vi "Tetra_RX-PROD_Setup.vi"() -> (0 "error out":errorcluster, 2 "Status":string)   [LabVIEW 2018]
uses:
  <vilib>/Utility/error.llb/DialogType.ctl
  Initialize References/Sequence Globals.vi
  Tetra_Globals.vi
  Infrastructure/Test Parameter Globals_1.0.0.vi
  Initialize References/Station References Global.vi
  Infrastructure/Test Result File Name Global.vi
  <vilib>/Utility/file.llb/Write Delimited Spreadsheet (DBL).vi
  <vilib>/Utility/error.llb/Error Cluster From Error Code.vi
  <vilib>/Utility/file.llb/Read Delimited Spreadsheet (string).vi
  <vilib>/Utility/file.llb/Write Delimited Spreadsheet (string).vi
  <vilib>/ErrorRing/Error Ring.xnode
  Instruments/PNA/lib functions/Agilent ENA Series.lvlib
  Instruments/Agilent N5232A PNA-L/Labview Driver/Keysight PNA Series/Keysight PNA Series.lvlib
  Instruments/Agilent PSG MXG Series/Agilent PSG MXG Series.lvlib
panel:
  in  "RevBTestBoard(t)":bool=TRUE
  out "RF_CAL_PATH(str)":string
  out "Capt_Rx_Data(t)":bool
  out "capt_dir":string
  out "Pmic_FwRev":string
  out "snic":string="#Family: 0x2D\n#Serial: 0x000036092740\r\n"
  out "rev":string="rdiv\r\n0)  sw3p6:   195 mA  3616 mV\r\n1)  sw5p5:    89 mA  5472 mV\r\n2) sw2p8a:   315 mA  2784 mV\r\n3) sw2p8b:   349 mA  2768 mV\r\n4)  sw2p4:  1458 mA  2288 mV\r\n5)  sw1p4:  1047 mA  1304 mV\r\n>"
  out "Tab Control":enum32{"Page 1", "Page 2", "Page 3", "Page 4"}(tab)
  in  "Setup Chip (T)":bool=TRUE
  in  "Setup Power Supply (T)":bool=TRUE
  in  "Setup PNA (T)":bool=TRUE
  in  "Kill Teraterm":bool=TRUE
  in  "Setup Gantry(t)":bool=TRUE
  out "FPGA_Booted":bool
  out "CAL_ADC(t)":bool
  out "Ping_Success":bool
  out "Success":bool
  out "COM PORT":string
  out "adccal":string
  out "fixed_if(t)":bool=TRUE
  out "Apply_FSPL":bool
  out "Use PS1-1":bool=TRUE
  out "Temp(t)":bool=TRUE
  out "FAST_DATA":bool
  out "IF_FREQ_MHZ":dbl caption="Delay Time (s)"
  out "MODE":string
  out "Text":refnum<vi>
  out "RF_POWER":dbl
  out "RF_FREQ":dbl
  out "REF_PWR":dbl
  out "REF_FREQ":dbl
  out "RX_GAIN":i32
  out "PS1-1(V)":dbl=3.0
  out "PS1-1(A)":dbl
  out "Array":dbl[][](array[numeric])
  out "RX_N_FREQ_LIST":dbl[](array[numeric])
  out "Temp Soak(min)":dbl caption="Delay Time (s)"
  out "Gantry_Z":dbl
  out "PORT":i16
  out "i_mon":string
  out "CMD":string
  out "fspl_cal_file":path
  out "PNA_STATE":string
  out "FSPL_CAL_FILE_DIR":path=path "C:/RageATE/Automated Tests/Tetra WAM/DVT/Cal Files/FSPL.csv"
  out "RF_CAL_PATH":path
  out "HORN_CAL_PATH":path
  out "NF_SPEC_FILE":path
  out "git log":string="#RageATE gitlog: commit 3f967c02fb9022fedaa326db1cba8dee33b37288\n#RageATE gitlog: Author: Rick-Rage <74794943+Rick-Rage@users.noreply.github.com>\n#RageATE gitlog: Date:   Tue Nov 23 14:33:10 2021 -0500\n#RageATE gitlog: This Computer Name : CRANES\r\n\r\n"
  out "TEMP":dbl=4.75
  out "Use PS1-2":bool=TRUE
  out "PS1-2(A)":dbl
  out "PS1-2(V)":dbl=1000000.0
  in  "error in (no error)":errorcluster
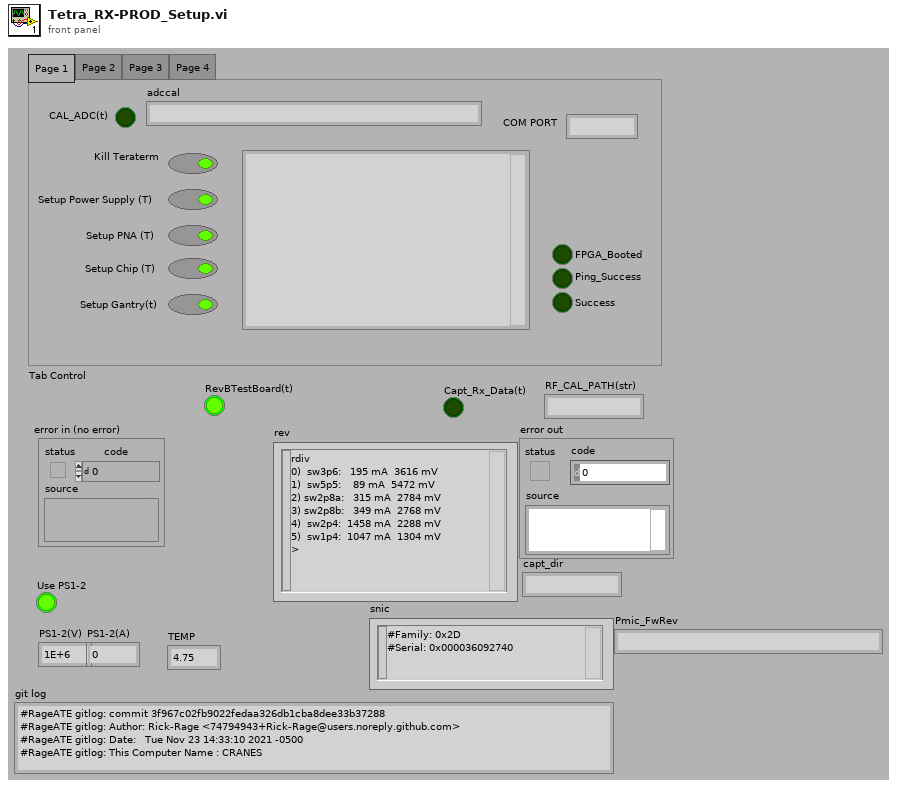
[diagram p1: front panel]
types:
  T1 = typedef "DialogType.ctl" = u16
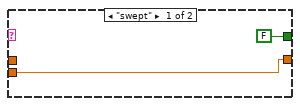
[diagram p4: hidden frame]
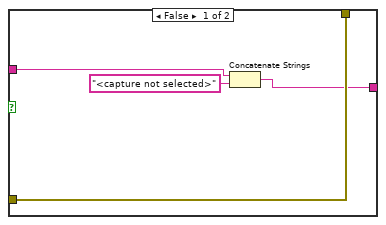
[diagram p5: hidden frame]
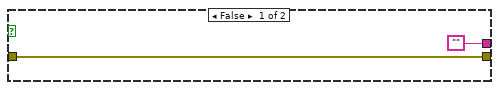
[diagram p6: hidden frame]
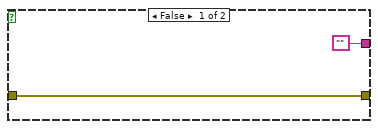
[diagram p7: hidden frame]
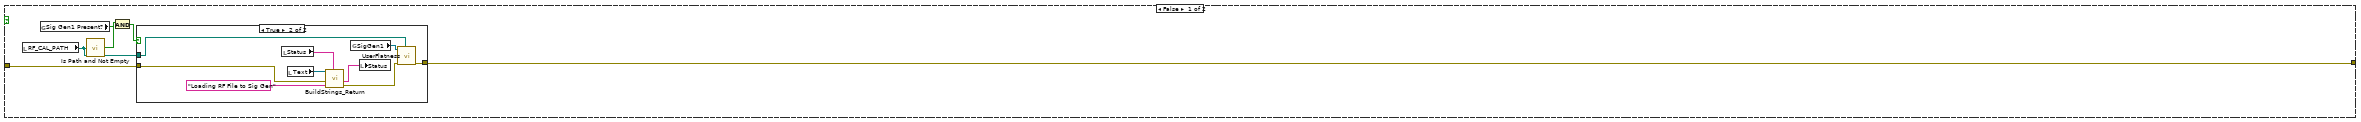
[diagram p8: hidden frame]
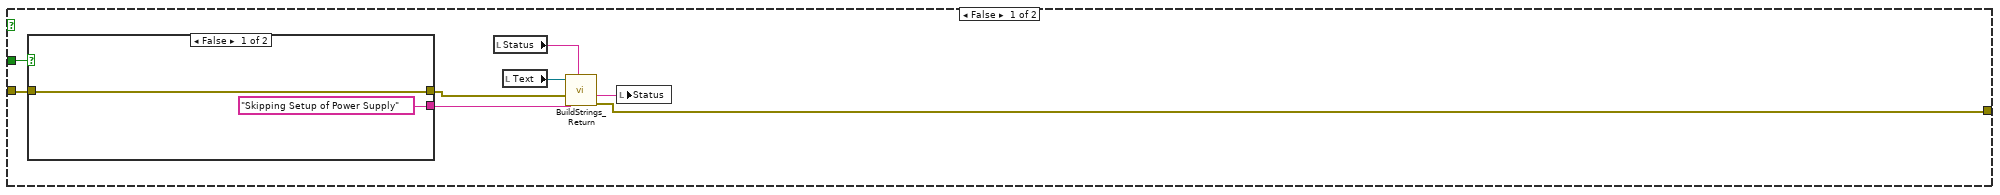
[diagram p15: hidden frame]
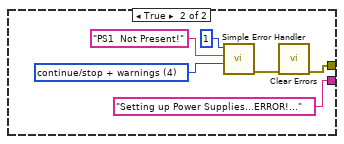
[diagram p16: hidden frame]
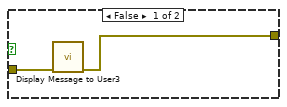
[diagram p18: hidden frame]
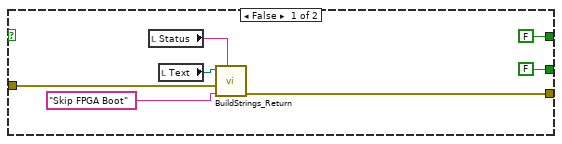
[diagram p20: hidden frame]
diagram:
  n1 = flat-sequence {
    tunnel: [w38] -> w18
    tunnel: w18 -> [w71]
    tunnel: [w70] -> w17
    tunnel: [w69] -> w16
    tunnel: [w67] -> w7
    tunnel: [w101] -> w9
    tunnel: w17 -> [w150]
    tunnel: w16 -> [w149]
    tunnel: w7 -> [w101]
    tunnel: w9 -> [w167]
    tunnel: [w177] -> w8
    tunnel: w8 -> [w229]
    tunnel: [w228] -> w14
    tunnel: w14 -> [w377]
    tunnel: [w376] -> w13
    tunnel: w13 -> [w385]
    tunnel: [w385] -> w1
    tunnel: [w387] -> w11
    tunnel: w1 -> [w386]
    tunnel: w11 -> [w473]
    tunnel: [w472] -> w4
    tunnel: [w510] -> w5
    tunnel: w4 -> [w509]
    tunnel: [w558] -> w6
    tunnel: w5 -> [w557]
    tunnel: w6 -> [w585]
    tunnel: [w584] -> w10
    tunnel: [w642] -> w19
    tunnel: w10 -> [w632]
    tunnel: [w794] -> w15
    tunnel: w19 -> [w788]
    tunnel: w15 -> [w838]
    tunnel: [w837] -> w3
    tunnel: w3 -> [w861]
    tunnel: [w860] -> w2
    tunnel: [w905] -> w12
    tunnel: w2 -> [w916]
    frame #0 {
      w28 = FALSE ("FPGA_Booted")
      # "Kill TeraTerm"
      n2 = flat-sequence {
        tunnel: [w57] -> w20
        tunnel: [w47] -> w21
        frame #0 {
          w54 = 0 items=["INPUT", "OUTPUT"] ("line index")
          # "C:\\RageATE\\Automated Tests\\Tetra WAM\\Support"
          n3 = global read "Sequence Globals.vi" "DevSupportPath"() -> (w44:path)
          n4 = Strip Path(path=w44) -> (stripped path=w43:path)  [unwired: 1 out]
          n5 = global read "Sequence Globals.vi" "AppSupportPath"() -> (w52:path)
          n6 = Build Path(base path=w43, name or relative path=path "Automated Tests/Tetra WAM/PRODUCTION/Test Benches" ("base path")) -> (appended path=w41:path)
          n7 = global read "Tetra_Globals.vi" "TestBench_ID"() -> (w45:string)
          n8 = global read "Sequence Globals.vi" "IsRuntime?"() -> (w40:bool)
          n9 = Build Path(base path=w41, name or relative path=w45) -> (appended path=w56:path)
          n10 = Concatenate Strings(w45, " Calibration Files" ("name or relative path")) -> (w46:string)
          n11 = Build Path(base path=w56, name or relative path=w46) -> (appended path=w53:path)
          n12 = Select(t=w52, s=w40, f=w53) -> (s? t:f=w48:path)
          n13 = call "FindMostRecentCalFile.vi"("DIR_IN"=w48, "Test Bench (for filename match)"=w45, "line index"=w54, "IsRuntime?"=w40) -> ("Success?(t)"=w50:bool, "cal_path_out"=w51:path)  [unwired: 9 in, 1 out]
          n14 = case shown="False" w50 {
            tunnel: [path "" ("appended path") w60] -> w57
            tunnel: w51 -> [_ w60]
            frame False {
              n15 = Two Button Dialog(message="There Are No INPUT cal files") -> ()  [unwired: 2 in, 1 out]
            }
            frame True {
            }
          }
          n16 = Build Path(base path=w48, name or relative path="FSPL.csv") -> (appended path=w47:path)
        }
      }
      n17 = global read "Sequence Globals.vi" "RageATE_Gitlog"() -> (→"git log":string)
      n18 = local write "RevBTestBoard(t)"("RevBTestBoard(t)") -> ()
      n19 = local write "CAL_ADC(t)"(w28) -> ()
      n20 = local write "Setup PNA (T)"("Setup PNA (T)") -> ()
      n21 = local write "Setup Gantry(t)"("Setup Gantry(t)") -> ()
      n22 = local write "Setup Chip (T)"("Setup Chip (T)") -> ()
      n23 = local write "Setup Power Supply (T)"("Setup Power Supply (T)") -> ()
      n24 = case shown="True" "Kill Teraterm" {
        tunnel: "error in (no error)" -> [w61 w63]
        tunnel: [w61 w62] -> w38
        tunnel: "taskkill /f /im ttermpro.exe" ("command line") -> [_ w65]
        frame False {
        }
        frame True {
          n25 = call <vilib>:"Clear Errors.vi"("error in (no error)"=w63) -> ("error out"=w64:errorcluster)  [unwired: 5 in, 1 out]
          n26 = call <vilib>:"System Exec.vi"("error in (no error)"=w64, "command line"=w65) -> ("error out"=w66:errorcluster)  [unwired: 6 in, 3 out]
          n27 = call "Time Delay2"("error in (no error)"=w66) -> ("error out"=w62:errorcluster)  [unwired: 10 in]
        }
      }
      n28 = Path To String(path=w20) -> (string=w26:string)
      n29 = Concatenate Strings("#RF_Cal_Path: " ("string"), w26) -> (→"RF_CAL_PATH(str)":string)
      "Success" <- FALSE ("Success")
      "Status" <- ""
      "adccal" <- ""
      "FPGA_Booted" <- w28
      "Ping_Success" <- w28
      "Tab Control" <- enum32{"Page 1", "Page 2", "Page 3", "Page 4"}."Page 1" ("Tab Control")
      "RF_CAL_PATH" <- w20
      "FSPL_CAL_FILE_DIR" <- w21
    }
    frame #1 {
      n30 = property on="Status" class="Str"(error in=w71) -> (error out=w67:errorcluster, "Text"=→"Text":refnum<vi>)  [unwired: 1 in, 1 out]
      n31 = global read "Test Parameter Globals_1.0.0.vi" "Input Constants Out"() -> (w70:string[])
      n32 = global read "Test Parameter Globals_1.0.0.vi" "Test Parameters"() -> (w69:string[][])
    }
    frame #2 {
      w140 = 0 ("disabled index (col)")
      # "PRODUCTION\\Test Benches\\Common"
      # "PRODUCTION\\Test Benches\\Common"
      # "C:\\RageATE\\Automated Tests\\Tetra WAM\\PRODUCTION\\Test Benches\\Common\\Horn_Gain_121322.csv"
      n33 = Index Array(array=w150, index #8=12 ("index"), index #9=14 ("index"), index #11=16 ("index"), index #16=24 ("index"), index #17=10 ("index")) -> (element #1=w129:string, element #2=w122:string, element #3=w92:string, element #4=→"MODE":string, element #5=w121:string, element #6=w116:string, element #7=w151:string, element #8=→"CMD":string, element #9=→"PNA_STATE":string, element #11=w88:string, element #12=w105:string, element #13=w104:string, element #14=w103:string, element #15=w100:string, element #16=w84:string, element #17=w96:string)  [unwired: 12 in, 1 out]
      n34 = call "StringToNumberControlWithBool.vi"("String In"=w96) -> ("NOT = 0"=→"Capt_Rx_Data(t)":bool)  [unwired: 7 in, 1 out]
      n35 = Index Array(array=w149, index (row) #1=0 ("disabled index (row)"), index (col) #1=w140, index (row) #2=3 ("index (row)"), index (col) #2=w140, index (row) #3=4 ("disabled index (row)"), index (col) #3=w140, index (row) #4=7 ("disabled index (row)"), index (col) #4=w140, index (row) #5=6 ("disabled index (row)"), index (col) #5=w140) -> (element #1=w143:string, element #2=w155:string, element #3=w154:string, element #4=w145:string, element #5=w138:string)
      n36 = call "StringToNumberControlWithBool.vi"("String In"=w151) -> ("Number Out"=→"Temp Soak(min)":dbl)  [unwired: 7 in, 1 out]
      n37 = call "StringToNumberControlWithBool.vi"("String In"=w104) -> ("NOT = 0"=→"FAST_DATA":bool)  [unwired: 7 in, 1 out]
      n38 = call "StringToNumberControlWithBool.vi"("String In"=w103) -> ("NOT = 0"=→"Apply_FSPL":bool)  [unwired: 7 in, 1 out]
      n39 = call "StringToNumberControlWithBool.vi"("String In"=w100) -> ("NOT = 0"=→"CAL_ADC(t)":bool)  [unwired: 7 in, 1 out]
      n40 = call "StringToNumberControlWithBool.vi"("String In"=w155) -> ("Number Out"=→"REF_PWR":dbl)  [unwired: 7 in, 1 out]
      n41 = call "StringToNumberControlWithBool.vi"("String In"=w154) -> ("Number Out"=→"RF_POWER":dbl)  [unwired: 7 in, 1 out]
      n42 = call "StringToNumberControlWithBool.vi"("String In"=w138) -> ("Number Out"=→"RX_GAIN":dbl)  [unwired: 7 in, 1 out]
      n43 = call "StringToNumberControlWithBool.vi"("String In"=w145) -> ("Number Out"=w111:dbl)  [unwired: 7 in, 1 out]
      "RF_FREQ" <- w111
      n44 = call "StringToNumberControlWithBool(x2).vi"("string"=w129) -> ("Num(2)"=→"PS1-1(A)":dbl, "Num"=→"PS1-1(V)":dbl, "NOT_0?"=→"Use PS1-1":bool)  [unwired: 4 in, 4 out]
      n45 = call "StringToNumberControlWithBool(x2).vi"("string"=w122) -> ("Num(2)"=→"PS1-2(A)":dbl, "Num"=→"PS1-2(V)":dbl, "NOT_0?"=→"Use PS1-2":bool)  [unwired: 4 in, 4 out]
      n46 = call "TempControlWithBool.vi"("INPUT"=w143) -> ("out"=→"TEMP":dbl, "Valid(t)"=w141:bool)  [unwired: 6 in, 1 out]
      "Temp(t)" <- w141
      n47 = call "StringToNumberControlWithBool(x2).vi"("string"=w121) -> ("Num(2)"=→"Gantry_Z":dbl, "Num"=→"PORT":dbl, "NOT_0(2)"=w119:bool, "NOT_0?"=w120:bool)  [unwired: 4 in, 3 out]
      n48 = call "StringToNumberControlWithBool(x2).vi"("string"=w116) -> ("Num(2)"=w113:dbl, "before substring"=w115:string)  [unwired: 4 in, 5 out]
      "IF_FREQ_MHZ" <- w113
      n49 = global write "Station References Global.vi" "Oven Present?"(w141) -> ()
      n50 = Or(x=w120, y=w119) -> (x .or. y?=w131:bool)
      n51 = call <vilib>:"Trim Whitespace.vi"("string"=w115) -> ("trimmed string"=w112:string)  [unwired: 1 in]
      n52 = Spreadsheet String To Array(delimiter (Tab)=";", format string="", spreadsheet string=w105, array type (2D Dbl)=dbl[] []) -> (array=w133:dbl[])
      "RX_N_FREQ_LIST" <- w133
      n53 = local write "Setup Gantry(t)"(w131) -> ()
      n54 = global write "Tetra_Globals.vi" "RX_N_FREQ_LIST"(w133) -> ()
      n55 = case shown="\"fixed\", Default" w112 {
        tunnel: [FALSE ("fixed_if(t)") TRUE ("fixed_if(t)")] -> w114
        tunnel: w113 -> [_ w164]
        tunnel: w111 -> [w157 w161]
        tunnel: [w157 w159] -> w110
        frame "swept" {
        }
        frame "fixed", Default {
          n56 = Divide(x=w164, y=1000.0) -> (x/y=w160:dbl)
          n57 = Add(x=w160, y=w161) -> (x+y=w163:dbl)
          n58 = Divide(x=w163, y=2.0) -> (x/y=w159:dbl)
        }
      }
      "REF_FREQ" <- w110
      "fixed_if(t)" <- w114
      n59 = global read "Sequence Globals.vi" "AppSupportPath"() -> (w81:path)
      n60 = global read "Sequence Globals.vi" "IsRuntime?"() -> (w83:bool)
      n61 = global read "Sequence Globals.vi" "DevSupportPath"() -> (w80:path)
      n62 = String To Path(string=w84) -> (path=w85:path)
      n63 = global read "Tetra_Globals.vi" "comport"() -> (w91:refnum<visa-resource-name>)
      n64 = Empty String/Path?(string/path=w92) -> (empty?=w94:bool)
      n65 = String To Path(string=w88) -> (path=w90:path)
      n66 = Strip Path(path=w85) -> (name=w76:string)  [unwired: 1 out]
      n67 = Strip Path(path=w80) -> (stripped path=w79:path)  [unwired: 1 out]
      n68 = Select(t=w91, s=w94, f=w92) -> (s? t:f=→"COM PORT":refnum<visa-resource-name>)
      n69 = Strip Path(path=w90) -> (name=w77:string)  [unwired: 1 out]
      n70 = Build Path(base path=w81, name or relative path=w76) -> (appended path=w86:path)
      n71 = Build Path(base path=w79, name or relative path="Automated Tests\\Tetra WAM\\PRODUCTION\\setup files") -> (appended path=w72:path)
      n72 = Build Path(base path=w72, name or relative path=w77) -> (appended path=w78:path)
      n73 = Build Path(base path=w81, name or relative path=w77) -> (appended path=w89:path)
      n74 = Select(t=w89, s=w83, f=w78) -> (s? t:f=→"HORN_CAL_PATH":path)
      n75 = Build Path(base path=w72, name or relative path=w76) -> (appended path=w75:path)
      n76 = Select(t=w86, s=w83, f=w75) -> (s? t:f=→"NF_SPEC_FILE":path)
    }
    frame #3 {
      # "Shut Off Equipments Power FOR ADC CAL"
      n77 = global read "Station References Global.vi" "PNA Present?"() -> (w176:bool)
      n78 = local read "CAL_ADC(t)"() -> (w171:bool)
      n79 = And(x=w176, y=w171) -> (x .and. y?=w172:bool)
      n80 = case shown="True" w172 {
        tunnel: [w199 w205] -> w178
        tunnel: w168 -> [w199 w207]
        tunnel: ["" w200] -> w173
        frame False {
        }
        frame True {
          w208 = 3 items=["HOLD", "CONT", "GROUP", "SINGLE"] ("Mode")
          w210 = 0 items=["OFF", "ON"] ("STATE(0=OFF)")
          n81 = global read "Station References Global.vi" "PNA"() -> (w214:refnum<visa-resource-name>)
          n82 = call "PNA_MAIN_RF_STATE.vi"("Session In"=w214, "error in"=w207, "RO(T)"=FALSE, "STATE(0=OFF)"=w210) -> ("Session Out"=w213:refnum<visa-resource-name>, "error out"=w212:errorcluster)  [unwired: 9 in, 1 out]
          n83 = call "PNA_SWEEP MODE.vi"("Mode"=w208, "Channel"=1, "error in (no error)"=w212, "VISA resource name"=w213) -> ("error out"=w206:errorcluster)  [unwired: 6 in, 1 out]
          n84 = local read "Status"() -> (w204:string)
          n85 = local read "Text"() -> (w202:refnum<vi>)
          n86 = call "BuildStrings_Return.vi"("seconds to wait"=1.0, "Input String"=w204, "New String"="Shutting Off PNA Power", "error in (no error)"=w206, "reference"=w202) -> ("error out"=w205:errorcluster, "concatenated string"=w200:string)  [unwired: 4 in, 1 out]
        }
      }
      n87 = flat-sequence {
        tunnel: w167 -> [w182]
        tunnel: [w181] -> w168
        frame #0 {
          n88 = local read "Capt_Rx_Data(t)"() -> (w179:bool)
          n89 = case shown="True" w179 {
            tunnel: [w184 w196] -> w183
            tunnel: w182 -> [w187 w191]
            tunnel: [w187 w190] -> w181
            tunnel: "#CaptureFileDirectory: " ("string") -> [w186 w189]
            frame False {
              n90 = Concatenate Strings(w186, "<capture not selected>" ("string")) -> (w184:string)
            }
            frame True {
              w188 = "'" ("string")
              # "For Header"
              n91 = global read "Test Result File Name Global.vi" "Test Results File Name"() -> (w197:path)
              n92 = Path To String(path=w197) -> (string=w195:string)
              n93 = Search and Replace String(input string=w195, search string=".csv", replace string="_RxCaptureFiles.zip" ("name or relative path"), error in=w191) -> (result string=w192:string, error out=w190:errorcluster)  [unwired: 4 in, 2 out]
              n94 = Concatenate Strings(w189, w188, w192, w188) -> (w196:string)
            }
          }
          "capt_dir" <- w183
        }
      }
      n95 = global read "Station References Global.vi" "Sig Gen1 Present?"() -> (w175:bool)
      n96 = local read "CAL_ADC(t)"() -> (w169:bool)
      n97 = local write "Status"(w173) -> ()
      n98 = And(x=w169, y=w175) -> (x .and. y?=w170:bool)
      n99 = case shown="True" w170 {
        tunnel: w178 -> [w216 w224]
        tunnel: [w216 w219] -> w177
        tunnel: ["" w218] -> w174
        frame False {
        }
        frame True {
          n100 = global read "Station References Global.vi" "SigGen1"() -> (w226:refnum<visa-resource-name>)
          n101 = call "VSG_SET_RF_STATE_1.00.vi"("RF ON/OFF (OFF)"=FALSE ("Enable RF Power (T: Enable)"), "error in"=w224, "Session In"=w226) -> ("error out"=w223:errorcluster)  [unwired: 6 in, 2 out]
          n102 = local read "Status"() -> (w217:string)
          n103 = local read "Text"() -> (w222:refnum<vi>)
          n104 = call "BuildStrings_Return.vi"("seconds to wait"=2.0, "Input String"=w217, "New String"="Shutting Off SG1 Power", "error in (no error)"=w223, "reference"=w222) -> ("error out"=w219:errorcluster, "concatenated string"=w218:string)  [unwired: 4 in, 1 out]
        }
      }
      n105 = local write "Status"(w174) -> ()
    }
    frame #4 {
      n106 = local read "Apply_FSPL"() -> (w227:bool)
      n107 = case shown="True" w227 {
        tunnel: w229 -> [w231 w253]
        tunnel: [w230 w252] -> w228
        frame False {
          n108 = local read "RF_CAL_PATH"() -> (w233:path)
          n109 = global read "Station References Global.vi" "Sig Gen1 Present?"() -> (w232:bool)
          n110 = call <vilib>:"Is Path and Not Empty.vi"("path"=w233) -> ("Is Path and Not Empty?"=w234:bool)  [unwired: 4 in]
          n111 = And(x=w234, y=w232) -> (x .and. y?=w235:bool)
          n112 = case shown="True" w235 {
            tunnel: w233 -> [_ w244]
            tunnel: w231 -> [w236 w240]
            tunnel: [w236 w238] -> w230
            frame False {
            }
            frame True {
              n113 = local read "Status"() -> (w237:string)
              n114 = local read "Text"() -> (w243:refnum<vi>)
              n115 = call "BuildStrings_Return.vi"("Input String"=w237, "New String"="Loading RF File to Sig Gen", "error in (no error)"=w240, "reference"=w243) -> ("error out"=w239:errorcluster, "concatenated string"=w242:string)  [unwired: 5 in, 1 out]
              n116 = global read "Station References Global.vi" "SigGen1"() -> (w245:refnum<visa-resource-name>)
              n117 = local write "Status"(w242) -> ()
              n118 = call "UserFlatness.vi"("cal file path (dialog if empty)"=w244, "error in (no error)"=w239, "Session In"=w245) -> ("error out"=w238:errorcluster)  [unwired: 6 in, 2 out]
            }
          }
        }
        frame True {
          n119 = flat-sequence {
            tunnel: w253 -> [w346]
            tunnel: [w347] -> w254
            tunnel: w254 -> [w362]
            tunnel: [w360] -> w247
            frame #0 {
              n120 = local read "RF_CAL_PATH"() -> (w344:path)
              n121 = call <vilib>:"Is Path and Not Empty.vi"("path"=w344) -> ("Is Path and Not Empty?"=w345:bool)  [unwired: 4 in]
              n122 = case shown="True" w345 {
                tunnel: [w348 w352] -> w347
                tunnel: w344 -> [_ w355]
                tunnel: w346 -> [w348 w350]
                frame False {
                }
                frame True {
                  n123 = call "GetCalData.vi"("Open new file T"=TRUE, "error in (no error)"=w350, "DeleteHeader(t)"=TRUE, "cal file path (dialog if empty)"=w355) -> ("error out"=w351:errorcluster, "array out"=w354:dbl[][])  [unwired: 2 in, 4 out]
                  n124 = global write "Tetra_Globals.vi" "RF_CAL"(w354) -> ()
                  n125 = local read "Status"() -> (w357:string)
                  n126 = local read "Text"() -> (w359:refnum<vi>)
                  n127 = call "BuildStrings_Return.vi"("Input String"=w357, "New String"="Reading RF Cal File...", "error in (no error)"=w351, "reference"=w359) -> ("error out"=w352:errorcluster, "concatenated string"=w358:string)  [unwired: 5 in, 1 out]
                  n128 = local write "Status"(w358) -> ()
                }
              }
            }
            frame #1 {
              n129 = local read "HORN_CAL_PATH"() -> (w361:path)
              n130 = Empty String/Path?(string/path=w361) -> (empty?=w363:bool)
              n131 = case shown="False" w363 {
                tunnel: w361 -> [w374 _]
                tunnel: w362 -> [w365 w375]
                tunnel: [w368 w375] -> w360
                frame False {
                  n132 = call "GetCalData.vi"("Open new file T"=TRUE, "error in (no error)"=w365, "DeleteHeader(t)"=FALSE, "cal file path (dialog if empty)"=w374) -> ("error out"=w366:errorcluster, "array out"=w373:dbl[][])  [unwired: 2 in, 4 out]
                  n133 = global write "Tetra_Globals.vi" "HORN_CAL"(w373) -> ()
                  n134 = local read "Status"() -> (w370:string)
                  n135 = local read "Text"() -> (w372:refnum<vi>)
                  n136 = call "BuildStrings_Return.vi"("Input String"=w370, "New String"="Reading Horn Cal File...", "error in (no error)"=w366, "reference"=w372) -> ("error out"=w368:errorcluster, "concatenated string"=w371:string)  [unwired: 5 in, 1 out]
                  n137 = local write "Status"(w371) -> ()
                }
                frame True {
                }
              }
            }
          }
          n138 = flat-sequence {
            tunnel: w247 -> [w256]
            tunnel: [w255] -> w246
            frame #0 {
              n139 = local read "NF_SPEC_FILE"() -> (w257:path)
              n140 = call <vilib>:"Is Path and Not Empty.vi"("path"=w257) -> ("Is Path and Not Empty?"=w258:bool)  [unwired: 4 in]
              n141 = case shown="True" w258 {
                tunnel: w257 -> [_ w265]
                tunnel: w256 -> [w259 w262]
                tunnel: [w259 w261] -> w255
                frame False {
                }
                frame True {
                  n142 = call "GetCalData.vi"("Open new file T"=TRUE, "error in (no error)"=w262, "DeleteHeader(t)"=TRUE, "cal file path (dialog if empty)"=w265) -> ("error out"=w261:errorcluster, "array out"=w263:dbl[][])  [unwired: 2 in, 4 out]
                  n143 = global write "Tetra_Globals.vi" "NF_MASK"(w263) -> ()
                }
              }
            }
          }
          n144 = flat-sequence {
            tunnel: [w324] -> w249
            tunnel: [w313] -> w250
            tunnel: w246 -> [w312]
            frame #0 {
              n145 = global read "Tetra_Globals.vi" "HORN_CAL"() -> (w325:dbl[][])
              n146 = for {
                tunnel: w325 -> [w341] mode=indexing
                tunnel: w312 -> [w340]
                tunnel: [w331] -> w322 mode=indexing
                tunnel: [w338] -> w323
                tunnel: [w335] -> w317 mode=indexing
                tunnel: [w332] -> w315 mode=indexing
                w330 = -1.0 ("x")
                w342 = u16 2 items=["Meter", "Feet", "Inches"] ("d(units)")
                w343 = u16 0 items=["GHz", "MHz"] ("f(units)")
                # "convert to mhz"
                n147 = Index Array(array=w341) -> (element #1=w337:dbl, element #2=w339:dbl)  [unwired: 2 in]
                n148 = local read "Gantry_Z"() -> (w334:dbl)
                n149 = Multiply(x=1000.0, y=w337) -> (x*y=w335:dbl)
                n150 = call "FSPL_CALC.vi"("f"=w337, "d"=w334, "error in"=w340, "Ant1 Gain (dB)"=w339, "f(units)"=w343, "d(units)"=w342) -> ("Corr(dB)"=w329:dbl, "fsl(dB)"=w333:dbl, "error out"=w338:errorcluster)  [unwired: 11 in]
                n151 = Multiply(x=w329, y=w330) -> (x*y=w331:dbl)
                n152 = Multiply(x=w330, y=w333) -> (x*y=w332:dbl)
              }
              n153 = local read "Gantry_Z"() -> (w316:dbl)
              n154 = Number To Fractional String(number=w316) -> (F-format string=w320:string)  [unwired: 3 in]
              n155 = local read "Status"() -> (w328:string)
              n156 = Concatenate Strings("Generating FSPL Table for Z = " ("New String"), w320, " inches" ("string")) -> (w319:string)
              n157 = local read "Text"() -> (w326:refnum<vi>)
              n158 = Build Array(w317, w322, w315) -> (w314:dbl[][])
              n159 = call "BuildStrings_Return.vi"("Input String"=w328, "New String"=w319, "error in (no error)"=w323, "reference"=w326) -> ("error out"=w324:errorcluster, "concatenated string"=w327:string)  [unwired: 5 in, 1 out]
              n160 = local write "Status"(w327) -> ()
              n161 = Transpose 2D Array(2D array=w314) -> (transposed array=w313:dbl[][])
              n162 = global write "Tetra_Globals.vi" "FSPL_CAL"(w313) -> ()
            }
          }
          n163 = flat-sequence {
            tunnel: w250 -> [w269]
            tunnel: w249 -> [w268]
            tunnel: [w267] -> w248
            frame #0 {
              n164 = for {
                tunnel: w269 -> [w279] mode=indexing
                tunnel: w268 -> [w277]
                tunnel: [w276] -> w267
                tunnel: [w273] -> w266 mode=indexing
                n165 = Index Array(array=w279) -> (element #1=w278:dbl, element #2=w272:dbl)  [unwired: 2 in]
                n166 = global read "Tetra_Globals.vi" "RF_CAL"() -> (w281:dbl[][])
                n167 = call "GetCalData.vi"("Open new file T"=FALSE, "Ary In"=w281, "error in (no error)"=w277, "RF Freq (MHz)"=w278, "DeleteHeader(t)"=FALSE) -> ("error out"=w276:errorcluster, "Ampl Out"=w271:dbl, "Cal Freq Out"=w274:dbl)  [unwired: 1 in, 3 out]
                n168 = Add(x=w271, y=w272) -> (x+y=w275:dbl)
                n169 = Build Array(w274, w275) -> (w273:dbl[])
              }
              "Array" <- w266
            }
          }
          n170 = flat-sequence {
            tunnel: [w307] -> w251
            tunnel: w248 -> [w297]
            frame #0 {
              n171 = local read "FSPL_CAL_FILE_DIR"() -> (w295:path)
              n172 = Path To String(path=w295) -> (string=w299:string)
              n173 = local read "Status"() -> (w304:string)
              n174 = Concatenate Strings("Writing Temp FSPL+Cal Correction File : " ("New String"), "\r", w299) -> (w301:string)
              n175 = local read "Text"() -> (w306:refnum<vi>)
              n176 = local read "Array"() -> (w296:dbl[][])
              n177 = call "BuildStrings_Return.vi"("Input String"=w304, "New String"=w301, "error in (no error)"=w297, "reference"=w306) -> ("error out"=w302:errorcluster, "concatenated string"=w305:string)  [unwired: 5 in, 1 out]
              n178 = local write "Status"(w305) -> ()
              n179 = global write "Tetra_Globals.vi" "RX_INPUT_OFFSET"(w296) -> ()
              n180 = call-poly <vilib>:"Write Delimited Spreadsheet.vi"("file path (dialog if empty)"=w295, "format (%.3f)"="%.3f", "2D data"=w296, "append to file? (new file:F)"=FALSE, "error in (no error)"=w302, "transpose? (no:F)"=FALSE, "delimiter (\\t)"="," ("delimiter (\\t)")) -> ("new file path (Not A Path if cancelled)"=→"fspl_cal_file":path, "error out"=w307:errorcluster)  [unwired: 7 in]
            }
          }
          n181 = flat-sequence {
            tunnel: w251 -> [w284]
            tunnel: [w283] -> w252
            frame #0 {
              n182 = global read "Station References Global.vi" "Sig Gen1 Present?"() -> (w282:bool)
              n183 = local read "Status"() -> (w287:string)
              n184 = local read "Text"() -> (w289:refnum<vi>)
              n185 = call "BuildStrings_Return.vi"("Input String"=w287, "New String"="Loading FSPL File to Sig Gen", "error in (no error)"=w284, "reference"=w289) -> ("error out"=w285:errorcluster, "concatenated string"=w288:string)  [unwired: 5 in, 1 out]
              n186 = local write "Status"(w288) -> ()
              n187 = case shown="True" w282 {
                tunnel: w285 -> [w290 w292]
                tunnel: [w290 w291] -> w283
                frame False {
                }
                frame True {
                  n188 = local read "fspl_cal_file"() -> (w293:path)
                  n189 = global read "Station References Global.vi" "SigGen1"() -> (w294:refnum<visa-resource-name>)
                  n190 = call "UserFlatness.vi"("cal file path (dialog if empty)"=w293, "error in (no error)"=w292, "Session In"=w294) -> ("error out"=w291:errorcluster)  [unwired: 6 in, 2 out]
                }
              }
            }
          }
        }
      }
    }
    frame #5 {
      n191 = global read "Station References Global.vi" "RF Switch Present?"() -> (w378:bool)
      n192 = case shown="True" w378 {
        tunnel: w377 -> [w379 w383]
        tunnel: [w379 w382] -> w376
        frame False {
        }
        frame True {
          n193 = global read "Station References Global.vi" "RF Switch"() -> (w384:refnum<visa-resource-name>)
          n194 = call "RfSwitch_WAM_ATE.vi"("VISA_IN"=w384, "error in"=w383, "Source"=enum16{"RFSM", "PNA"}."PNA", "T/R"=enum16{"TX", "RX"}."RX") -> ("error out"=w382:errorcluster)  [unwired: 10 in, 1 out]
        }
      }
    }
    frame #6 {
    }
    frame #7 {
      n195 = local read "Setup Power Supply (T)"() -> (w388:bool)
      n196 = global read "Station References Global.vi" "PS1 Present?"() -> (w390:bool)
      n197 = And(x=w390, y=w388) -> (x .and. y?=w389:bool)
      n198 = case shown="True" w389 {
        tunnel: [w392 w409] -> w387
        tunnel: w388 -> [w398 _]
        tunnel: w386 -> [w391 w408]
        frame False {
          n199 = case shown="False" w398 {
            tunnel: [w399 w402] -> w393
            tunnel: ["Skipping Setup of Power Supply" "Setting up Power Supplies...ERROR!..."] -> w394
            tunnel: w391 -> [w399 _]
            frame False {
            }
            frame True {
              w404 = T1 4 items=["no dialog", "OK message", "continue or stop message", "OK message + warnings", "continue/stop + warnings"] ("type of dialog (OK msg:1)")
              n200 = call <vilib>:"Simple Error Handler.vi"("error code (no error:0)"=1, "error source (\" \")"="PS1  Not Present!" ("error source (\" \")"), "type of dialog (OK msg:1)"=w404) -> ("error out"=w403:errorcluster)  [unwired: 2 in, 4 out]
              n201 = call <vilib>:"Clear Errors.vi"("error in (no error)"=w403) -> ("error out"=w402:errorcluster)  [unwired: 5 in, 1 out]
            }
          }
          n202 = local read "Status"() -> (w395:string)
          n203 = local read "Text"() -> (w397:refnum<vi>)
          n204 = call "BuildStrings_Return.vi"("Input String"=w395, "New String"=w394, "error in (no error)"=w393, "reference"=w397) -> ("error out"=w392:errorcluster, "concatenated string"=w396:string)  [unwired: 5 in, 1 out]
          n205 = local write "Status"(w396) -> ()
        }
        frame True {
          n206 = call "Prompt User for Input"("Enable"=FALSE, "error in (no error)"=w408) -> ("error out"=w412:errorcluster)  [unwired: 16 in, 1 out]
          n207 = local read "Status"() -> (w414:string)
          n208 = local read "Text"() -> (w413:refnum<vi>)
          n209 = call "BuildStrings_Return.vi"("Input String"=w414, "New String"="Setting up the Power Supplies...", "error in (no error)"=w412, "reference"=w413) -> ("error out"=w415:errorcluster, "concatenated string"=w410:string)  [unwired: 5 in, 1 out]
          n210 = local write "Status"(w410) -> ()
          n211 = for {
            N: 2 -> [w422]
            tunnel: w410 -> [w433]
            shift-right: [w425] -> w409
            shift-left: w415 -> [w437]
            i -> [w424]
            stop <- w427 continue-if-true
            n212 = stacked-sequence {
              tunnel: w437 -> [w471]
              tunnel: [w470] -> w434
              frame #0 {
                w455 = "PS1" ("SEL_PS")
                # "Conf I/V lim"
                n213 = local read "PS1-2(V)"() -> (w466:dbl)
                n214 = local read "PS1-2(A)"() -> (w467:dbl)
                n215 = local read "Text"() -> (w458:refnum<vi>)
                n216 = local read "PS1-1(A)"() -> (w468:dbl)
                n217 = local read "PS1-1(V)"() -> (w465:dbl)
                n218 = property class="Txt"(reference=w458, error in=w471, "Scroll Position"=i16 -1) -> (error out=w456:errorcluster)  [unwired: 1 out]
                n219 = global read "Station References Global.vi" "PS1"() -> (w469:refnum<visa-resource-name>)
                n220 = Build Array(w468, w467, 1.0 ("element")) -> (w461:dbl[])
                n221 = Build Array(w465, w466, 12.0 ("element")) -> (w460:dbl[])
                n222 = call "PS_SETUP_V-I-EN.vi"("VISA resource name"=w469, "SEL_PS"=w455, "error in (no error)"=w456, "Use Channel"=bool[] [FALSE, FALSE, FALSE, FALSE], "Current Lim"=w461, "Voltage Set"=w460) -> ("VISA resource name out"=w459:refnum<visa-resource-name>, "error out"=w463:errorcluster)  [unwired: 8 in]
                n223 = call "Time Delay5"("error in (no error)"=w463) -> ("error out"=w454:errorcluster)  [unwired: 10 in]
                n224 = call "PS_SETUP_V-I-EN.vi"("VISA resource name"=w459, "SEL_PS"=w455, "error in (no error)"=w454, "Use Channel"=bool[] [TRUE, FALSE, FALSE, FALSE], "Current Lim"=w461, "Voltage Set"=w460) -> ("error out"=w470:errorcluster)  [unwired: 8 in, 1 out]
              }
            }
            n225 = Increment(x=w424) -> (x+1=w423:i32)
            n226 = local read "Text"() -> (w436:refnum<vi>)
            n227 = call "BuildStrings_Return.vi"("Input String"=w433, "New String"="Power Supplies ON!", "error in (no error)"=w434, "reference"=w436) -> ("error out"=w432:errorcluster, "concatenated string"=w431:string)  [unwired: 5 in, 1 out]
            n228 = local write "Status"(w431) -> ()
            n229 = Equal?(x=w422, y=w423) -> (x = y?=w421:bool)
            n230 = control-ref of="Text"() -> (w429:refnum<vi>)
            n231 = control-ref of="Status"() -> (w430:refnum<vi>)
            n232 = call "DcPreBootTest.vi"("String in"=w430, "lsl/hsl limit"=dbl[] [0.01, 0.6], "reference in"=w429, "concatenated string"=w431, "error in (no error)"=w432, "seconds to wait"=1.0) -> ("DcLow?(t= low)"=w428:bool, "concatenated stringout"=w418:string, "FlagDC?(t)"=w427:bool, "error out"=w426:errorcluster)  [unwired: 6 in]
            n233 = local write "Status"(w418) -> ()
            n234 = global read "Station References Global.vi" "PS1"() -> (w420:refnum<visa-resource-name>)
            n235 = case shown="True" w428 {
              selector: w428 -> [_ w442]
              tunnel: w426 -> [w438 w444]
              tunnel: [w438 w443] -> w425
              tunnel: w421 -> [_ w439]
              tunnel: w420 -> [_ w440]
              frame False {
              }
              frame True {
                n236 = And(x=w442, y=w439) -> (x .and. y?=w441:bool)
                n237 = case shown="True" w441 {
                  tunnel: w444 -> [w446 w450]
                  tunnel: [w445 w447] -> w443
                  tunnel: w440 -> [_ w451]
                  frame False {
                    n238 = call "Display Message to User3"("error in (no error)"=w446) -> ("error out"=w445:errorcluster)  [unwired: 9 in, 1 out]
                  }
                  frame True {
                    n239 = call "PS_SETUP_V-I-EN.vi"("VISA resource name"=w451, "error in (no error)"=w450, "Use Channel"=bool[] [FALSE, FALSE, FALSE, FALSE]) -> ("error out"=w448:errorcluster)  [unwired: 11 in, 1 out]
                    n240 = call "Display Message to User4"("error in (no error)"=w448) -> ("error out"=w447:errorcluster)  [unwired: 9 in, 1 out]
                    n241 = invoke class="VI" method="FP.Close"(error in=w447) -> ()  [unwired: 2 in, 3 out]
                  }
                }
              }
            }
          }
        }
      }
    }
    frame #8 {
      n242 = flat-sequence {
        tunnel: w473 -> [w479]
        tunnel: [w475] -> w472
        frame #0 {
          n243 = local read "Setup Chip (T)"() -> (w480:bool)
          n244 = case shown="True" w480 {
            selector: w480 -> [_ w496]
            tunnel: [FALSE ("Success") w508] -> w474
            tunnel: [w488 w495] -> w478
            tunnel: w479 -> [w489 w499]
            tunnel: [FALSE w496] -> w476
            frame False {
              n245 = local read "Status"() -> (w491:string)
              n246 = local read "Text"() -> (w492:refnum<vi>)
              n247 = call "BuildStrings_Return.vi"("Input String"=w491, "New String"="Skip FPGA Boot", "error in (no error)"=w489, "reference"=w492) -> ("error out"=w488:errorcluster)  [unwired: 5 in, 2 out]
            }
            frame True {
              n248 = local read "Status"() -> (w503:string)
              n249 = local read "Text"() -> (w502:refnum<vi>)
              n250 = call "BuildStrings_Return.vi"("seconds to wait"=8.5, "Input String"=w503, "New String"="Booting up FPGA...\nTakes up to 15sec..." ("Delay text ..."), "error in (no error)"=w499, "reference"=w502) -> ("error out"=w498:errorcluster, "concatenated string"=w497:string)  [unwired: 4 in, 1 out]
              n251 = local read "COM PORT"() -> (w505:string)
              n252 = local write "Status"(w497) -> ()
              n253 = call "Tetra Serial.vi"("COMPORT"=w505, "error in (no error)"=w498, "Command"="", "Open Ser(t)"=TRUE, "Close Ser(t)"=FALSE) -> ("Success"=w508:bool, "error out"=w495:errorcluster)  [unwired: 6 in, 3 out]
            }
          }
          n254 = And(x=w474, y=w476) -> (x .and. y?=w477:bool)
          n255 = local write "FPGA_Booted"(w474) -> ()
          n256 = case shown="True" w477 {
            tunnel: w478 -> [w481 w486]
            tunnel: [w481 w482] -> w475
            frame False {
            }
            frame True {
              n257 = local read "Status"() -> (w485:string)
              n258 = local read "Text"() -> (w487:refnum<vi>)
              n259 = call "BuildStrings_Return.vi"("Input String"=w485, "New String"="FPGA Success!!", "error in (no error)"=w486, "reference"=w487) -> ("error out"=w482:errorcluster, "concatenated string"=w483:string)  [unwired: 5 in, 1 out]
              n260 = local write "Status"(w483) -> ()
            }
          }
        }
      }
    }
    frame #9 {
      n261 = global read "Station References Global.vi" "Oven Present?"() -> (w511:bool)
      n262 = local read "Temp(t)"() -> (w512:bool)
      n263 = And(x=w512, y=w511) -> (x .and. y?=w513:bool)
      n264 = case shown="True" w513 {
        tunnel: w512 -> [w519 _]
        tunnel: [w517 w539] -> w510
        tunnel: w509 -> [w514 w552]
        frame False {
          n265 = call "Display Message to User"("error in (no error)"=w514, "Enable"=w519) -> ("error out"=w516:errorcluster, "Cancel"=w518:bool)  [unwired: 8 in]
          n266 = Stop(stop? (T)=w518) -> ()
          n267 = case shown="False" w518 {
            tunnel: [w525 w527] -> w515
            tunnel: [w524 w528] -> w517
            tunnel: w516 -> [w523 w528]
            frame False {
              n268 = local read "Status"() -> (w521:string)
              n269 = local read "Text"() -> (w522:refnum<vi>)
              n270 = call "BuildStrings_Return.vi"("Input String"=w521, "New String"="Skipping Setting Up Temperature...", "error in (no error)"=w523, "reference"=w522) -> ("error out"=w524:errorcluster, "concatenated string"=w525:string)  [unwired: 5 in, 1 out]
            }
            frame True {
              n271 = local read "Status"() -> (w527:string)
            }
          }
          n272 = disable-structure shown="Disabled" {
            frame Disabled {
              n273 = global write "Station References Global.vi" "Oven Present?"(FALSE ("Oven Present?")) -> ()
            }
            frame Enabled {
            }
          }
          n274 = local write "Status"(w515) -> ()
        }
        frame True {
          w547 = u16 10 items=["READ ONLY"=0, "AUTO"=10, "OFF"=62, "MAN"=54] ("MODE")
          n275 = local read "Temp Soak(min)"() -> (w535:dbl)
          n276 = local read "TEMP"() -> (w542:dbl)
          n277 = Number To Fractional String(number=w542) -> (F-format string=w541:string)  [unwired: 3 in]
          n278 = Number To Fractional String(number=w535) -> (F-format string=w533:string)  [unwired: 3 in]
          n279 = Concatenate Strings("Setting Temp Plate to  ", w541, " °C" ("string"), " and Soak for " ("string"), w533, " min" ("string")) -> (w543:string)
          n280 = local read "Status"() -> (w544:string)
          n281 = local read "Text"() -> (w545:refnum<vi>)
          n282 = call "BuildStrings_Return.vi"("Input String"=w544, "New String"=w543, "error in (no error)"=w552, "reference"=w545) -> ("error out"=w549:errorcluster, "concatenated string"=w530:string, "reference out"=w537:refnum<vi>)  [unwired: 5 in]
          n283 = local write "Status"(w530) -> ()
          n284 = global read "Station References Global.vi" "Oven"() -> (w550:refnum<visa-resource-name>)
          n285 = call "PM9_TCP_MODE.vi"("VISA"=w550, "error in (no error)"=w549, "MODE"=w547, "Close tcp(t)"=TRUE) -> ("visa out"=w546:refnum<visa-resource-name>, "error out"=w551:errorcluster)  [unwired: 8 in, 2 out]
          n286 = local read "TEMP"() -> (w555:dbl)
          n287 = call "PM9 Set Temp and Wait.vi"("VISA"=w546, "Error In"=w551, "Accuracy +/-"=1.0, "Set Point"=w555, "Min (-1 for cont.)"=0.0, "close session(t)"=TRUE) -> ("error out"=w538:errorcluster)  [unwired: 10 in, 3 out]
          n288 = call "BuildStrings_Return.vi"("Input String"=w530, "New String"="Temp Set and Soak Complete!", "error in (no error)"=w538, "reference"=w537) -> ("error out"=w539:errorcluster, "concatenated string"=w536:string)  [unwired: 5 in, 1 out]
          n289 = local write "Status"(w536) -> ()
        }
      }
    }
    frame #10 {
      n290 = flat-sequence {
        tunnel: [w562] -> w558
        tunnel: w557 -> [w561]
        frame #0 {
          n291 = local read "COM PORT"() -> (w559:string)
          n292 = local read "CAL_ADC(t)"() -> (w563:bool)
          n293 = case shown="False" w563 {
            tunnel: w561 -> [w565 w575]
            tunnel: [w565 w569] -> w562
            tunnel: ["#NotSelected" ("cal_adc_delay") w567] -> w560
            tunnel: w559 -> [_ w579]
            frame False {
            }
            frame True {
              n294 = local read "Status"() -> (w577:string)
              n295 = local read "Text"() -> (w576:refnum<vi>)
              n296 = call "BuildStrings_Return.vi"("Input String"=w577, "New String"="Running ADC Cal...", "error in (no error)"=w575, "reference"=w576) -> ("error out"=w574:errorcluster, "concatenated string"=w568:string, "reference out"=w571:refnum<vi>)  [unwired: 5 in]
              n297 = call "Tetra_CalAdc.vi"("COMPORT"=w579, "error in (no error)"=w574) -> ("cal_adc_mag"=w572:string, "cal_adc_delay"=w573:string, "error out"=w570:errorcluster)  [unwired: 12 in, 3 out]
              n298 = Concatenate Strings("#" ("string"), w573, w572) -> (w567:string)
              n299 = call "BuildStrings_Return.vi"("Input String"=w568, "New String"=w567, "error in (no error)"=w570, "reference"=w571) -> ("error out"=w569:errorcluster, "concatenated string"=w566:string)  [unwired: 5 in, 1 out]
              n300 = local write "Status"(w566) -> ()
            }
          }
          n301 = local write "adccal"(w560) -> ()
        }
      }
    }
    frame #11 {
      n302 = local read "FAST_DATA"() -> (w586:bool)
      n303 = case shown="True" w586 {
        tunnel: w585 -> [w588 w591]
        tunnel: [w588 w590] -> w584
        tunnel: [TRUE ("OK") w589] -> w583
        frame False {
        }
        frame True {
          n304 = stacked-sequence {
            tunnel: [w594] -> w590
            tunnel: w591 -> [w592]
            tunnel: [w593] -> w589
            frame #0 {
              n305 = for {
                N: 2 -> [_]
                shift-right: [w601] -> w594
                shift-left: w592 -> [w605]
                tunnel: [w597] -> w593
                stop <- w597 stop-if-true
                n306 = local read "Status"() -> (w606:string)
                n307 = local read "Text"() -> (w608:refnum<vi>)
                n308 = call "BuildStrings_Return.vi"("seconds to wait"=1.0, "Input String"=w606, "New String"="Checking IP Address: 169.254.70.191, for Fast RxData", "error in (no error)"=w605, "reference"=w608) -> ("error out"=w602:errorcluster, "concatenated string"=w604:string)  [unwired: 4 in, 1 out]
                n309 = local write "Status"(w604) -> ()
                n310 = call "PingCmdLine.vi"("error in (no error)"=w602, "IP Address"="169.254.70.191" ("IP_ADDR")) -> ("error out"=w603:errorcluster, "Match?(t)"=w596:bool, "Ip_out"=w600:string)  [unwired: 7 in]
                n311 = case shown="True" w596 {
                  selector: w596 -> [w609 _]
                  tunnel: w603 -> [w614 w626]
                  tunnel: [w611 w625] -> w601
                  tunnel: w600 -> [w613 w623]
                  tunnel: [w610 TRUE] -> w597
                  frame False {
                    n312 = Concatenate Strings("Failed to Connect to " ("New String"), w613, "Check Address and Connections" ("string")) -> (w617:string)
                    n313 = local read "Status"() -> (w619:string)
                    n314 = local read "Text"() -> (w618:refnum<vi>)
                    n315 = call "BuildStrings_Return.vi"("Input String"=w619, "New String"=w617, "error in (no error)"=w614, "reference"=w618) -> ("error out"=w612:errorcluster, "concatenated string"=w620:string)  [unwired: 5 in, 1 out]
                    n316 = local write "Status"(w620) -> ()
                    n317 = call "Prompt User for Input2"("Enable"=w609, "error in (no error)"=w612) -> ("OK"=w610:bool, "error out"=w611:errorcluster)  [unwired: 16 in]
                  }
                  frame True {
                    n318 = Concatenate Strings(w623, "  Connected ..Success!!" ("New String")) -> (w624:string)
                    n319 = local read "Status"() -> (w628:string)
                    n320 = local read "Text"() -> (w627:refnum<vi>)
                    n321 = call "BuildStrings_Return.vi"("Input String"=w628, "New String"=w624, "error in (no error)"=w626, "reference"=w627) -> ("error out"=w625:errorcluster, "concatenated string"=w629:string)  [unwired: 5 in, 1 out]
                    n322 = local write "Status"(w629) -> ()
                  }
                }
                n323 = local write "Ping_Success"(w597) -> ()
              }
            }
          }
        }
      }
      n324 = local read "FPGA_Booted"() -> (w581:bool)
      n325 = And(x=w581, y=w583) -> (x .and. y?=w582:bool)
      n326 = local write "Success"(w582) -> ()
    }
    frame #12 {
      n327 = global read "Tetra_Globals.vi" "RevC(t)"() -> (w630:bool)
      n328 = case shown="True" w630 {
        tunnel: [w649 w655] -> w633
        tunnel: w632 -> [w649 w654]
        tunnel: ["#IMON RESULT : -1 " ("string") w652] -> w631
        frame False {
        }
        frame True {
          n329 = control-ref of="Text"() -> (w656:refnum<vi>)
          n330 = local read "COM PORT"() -> (w650:string)
          n331 = control-ref of="Status"() -> (w657:refnum<vi>)
          n332 = call "WAM-DC-HealthCheck.vi"("COMPORT"=w650, "error in (no error)"=w654, "reference in"=w657, "LVObjectRefNum in"=w656) -> ("error out"=w655:errorcluster, "i_mon"=w653:string)  [unwired: 5 in, 1 out]
          n333 = Concatenate Strings("#IMON_RESULT: " ("string"), w653) -> (w652:string)
        }
      }
      "i_mon" <- w631
      n334 = local read "Setup Chip (T)"() -> (w638:bool)
      n335 = local read "Success"() -> (w634:bool)
      n336 = And(x=w638, y=w634) -> (x .and. y?=w639:bool)
      n337 = case shown="True" w639 {
        selector: w639 -> [w685 w720]
        tunnel: w633 -> [w686 w704]
        tunnel: [w686 w699] -> w646
        tunnel: [w685 w720] -> w647
        frame False {
        }
        frame True {
          n338 = local read "MODE"() -> (w706:string)
          n339 = case shown="\"1\"" w706 {
            tunnel: ["" ";wr reg 0x04 1032" ("string")] -> w707
            tunnel: w704 -> [w772 w780]
            tunnel: [w773 w779] -> w703
            frame "0", Default {
              n340 = local read "Status"() -> (w777:string)
              n341 = local read "Text"() -> (w776:refnum<vi>)
              n342 = call "BuildStrings_Return.vi"("Input String"=w777, "New String"="Setting Mode to Manual", "error in (no error)"=w772, "reference"=w776) -> ("error out"=w773:errorcluster, "concatenated string"=w775:string)  [unwired: 5 in, 1 out]
              n343 = local write "Status"(w775) -> ()
            }
            frame "1" {
              n344 = local read "Status"() -> (w784:string)
              n345 = local read "Text"() -> (w783:refnum<vi>)
              n346 = call "BuildStrings_Return.vi"("Input String"=w784, "New String"="Setting Mode to Auto", "error in (no error)"=w780, "reference"=w783) -> ("error out"=w779:errorcluster, "concatenated string"=w782:string)  [unwired: 5 in, 1 out]
              n347 = local write "Status"(w782) -> ()
            }
          }
          n348 = local read "CMD"() -> (w700:string)
          n349 = Empty String/Path?(string/path=w700) -> (empty?=w701:bool)
          n350 = case shown="False" w701 {
            tunnel: [w746 ""] -> w702
            tunnel: w700 -> [w745 _]
            frame False {
              n351 = Concatenate Strings(";" ("string"), w745) -> (w746:string)
            }
            frame True {
            }
          }
          n352 = local read "COM PORT"() -> (w687:string)
          n353 = Concatenate Strings("rxdata real" ("Command ( ; seperation)"), w707, w702) -> (w708:string)
          n354 = global read "Tetra_Globals.vi" "BarCodeESN"() -> (w688:string)
          n355 = call "SerRW-Array.vi"("COMPORT"=w687, "error in (no error)"=w703, "Command ( ; seperation)"=w708) -> ("comport"=w711:refnum<visa-resource-name>, "error out"=w710:errorcluster)  [unwired: 6 in, 5 out]
          n356 = call "Tetra_Rev.vi"("COMPORT"=w711, "error in (no error)"=w710) -> ("rev"=→"rev":string, "comport"=w718:refnum<visa-resource-name>, "error out"=w717:errorcluster)  [unwired: 9 in, 2 out]
          n357 = call "Tetra_ReadESN.vi"("COMPORT"=w718, "BC_Esn"=w688, "error in (no error)"=w717) -> ("read"=→"snic":string, "comport"=w692:refnum<visa-resource-name>, "esn"=w714:string, "error out"=w694:errorcluster)  [unwired: 8 in, 1 out]
          n358 = global write "Tetra_Globals.vi" "ESN"(w714) -> ()
          n359 = call "ESNLookup.vi"("ESN"=w714, "error in"=w694) -> ("error out"=w693:errorcluster)  [unwired: 7 in, 2 out]
          n360 = call "UCD_Device-Info.vi"("COMPORT"=w692, "error in (no error)"=w693) -> ("Pmic_FwRev"=→"Pmic_FwRev":string, "comport"=w691:refnum<visa-resource-name>, "error out"=w690:errorcluster)  [unwired: 10 in, 1 out]
          n361 = local read "Status"() -> (w712:string)
          n362 = local read "Text"() -> (w713:refnum<vi>)
          n363 = local read "RX_GAIN"() -> (w715:i32)
          n364 = call "BuildStrings_Return.vi"("Input String"=w712, "error in (no error)"=w690, "reference"=w713) -> ("error out"=w696:errorcluster, "concatenated string"=w695:string)  [unwired: 6 in, 1 out]
          n365 = local read "MODE"() -> (w705:string)
          n366 = local write "Status"(w695) -> ()
          n367 = case shown="\"0\", Default" w705 {
            tunnel: [w752 w769] -> w698
            tunnel: w691 -> [w751 w771]
            tunnel: w715 -> [w750 _]
            tunnel: w696 -> [w749 w770]
            frame "0", Default {
              n368 = case shown="0.." w750 {
                tunnel: w749 -> [w754 w760]
                tunnel: [w753 w759] -> w752
                tunnel: w751 -> [w755 w757]
                frame -1, Default {
                  n369 = VISA Close(VISA resource name=w755, error in (no error)=w754) -> (error out=w753:errorcluster)
                }
                frame 0.. {
                  n370 = global read "Tetra_Globals.vi" "RevC(t)"() -> (w756:bool)
                  n371 = for {
                    tunnel: w757 -> [w767]
                    tunnel: w760 -> [w766]
                    tunnel: [w765] -> w759
                    tunnel: i32[] [1, 3, 5, 7] -> [w764] mode=indexing
                    tunnel: [w763] -> _
                    tunnel: w756 -> [w761]
                    n372 = call "Tetra_RxGain.vi"("COMPORT"=w767, "error in (no error)"=w766, "RXPORT(num)"=w764, "Close Ser(t)"=TRUE, "GAIN(code)"=0, "REVC(T)"=w761) -> ("comport"=w763:refnum<visa-resource-name>, "error out"=w765:errorcluster)  [unwired: 9 in, 3 out]
                  }
                }
              }
            }
            frame "1" {
              n373 = VISA Close(VISA resource name=w771, error in (no error)=w770) -> (error out=w769:errorcluster)
            }
          }
          n374 = local read "FAST_DATA"() -> (w697:bool)
          n375 = case shown="True" w697 {
            tunnel: [w721 w731] -> w699
            tunnel: w698 -> [w721 w728]
            frame False {
            }
            frame True {
              w723 = TRUE  # Close Serial(T)
              w722 = TRUE  # ExeCommands(T)
              w724 = 0 items=["CW", "DYNAMIC"] ("Mode Select")
              n376 = global read "Tetra_Globals.vi" "RevC(t)"() -> (w726:bool)
              n377 = local read "Status"() -> (w735:string)
              n378 = local read "Text"() -> (w733:refnum<vi>)
              n379 = call "BuildStrings_Return.vi"("Input String"=w735, "New String"="Running AM_Init for Fast Data", "error in (no error)"=w728, "reference"=w733) -> ("error out"=w729:errorcluster, "concatenated string"=w732:string)  [unwired: 5 in, 1 out]
              n380 = local write "Status"(w732) -> ()
              n381 = local read "COM PORT"() -> (w725:string)
              n382 = call "PingTestBoard(LC).vi"("COMPORT"=w725, "error in (no error)"=w729, "Mode Select"=w724, "Close Serial(T)"=w723, "ExeCommands(T)"=w722, "RevC(t)"=w726) -> ("OK?(t)"=w727:bool, "error out"=w730:errorcluster)  [unwired: 7 in, 5 out]
              n383 = case shown="True" w727 {
                tunnel: w730 -> [w738 w743]
                tunnel: [w736 w744] -> w731
                frame False {
                  n384 = call "Display Message to User2"("error in (no error)"=w738, "Enable"=TRUE) -> ()  [unwired: 8 in, 2 out]
                  n385 = xnode "Error Ring"() -> ("error out"=w736:errorcluster)
                }
                frame True {
                  n386 = call <vilib>:"Clear Errors.vi"("error in (no error)"=w743) -> ("error out"=w744:errorcluster)  [unwired: 5 in, 1 out]
                }
              }
            }
          }
        }
      }
      n387 = And(x=w647, y=FALSE) -> (x .and. y?=w645:bool)
      n388 = case shown="False" w645 {
        tunnel: w646 -> [w658 w684]
        tunnel: [w659 w684] -> w643
        frame False {
          n389 = flat-sequence {
            tunnel: [w677] -> w659
            tunnel: w658 -> [w665]
            frame #0 {
              w660 = "\r\n"
              n390 = local read "RF_CAL_PATH(str)"() -> (w661:string)
              n391 = local read "git log"() -> (w668:string)
              n392 = local read "capt_dir"() -> (w662:string)
              n393 = global read "Test Result File Name Global.vi" "Test Results File Name"() -> (w663:path)
              n394 = local read "Pmic_FwRev"() -> (w671:string)
              n395 = global read "Test Parameter Globals_1.0.0.vi" "BarCodeInfo"() -> (w674:string)
              n396 = local read "rev"() -> (w673:string)
              n397 = local read "snic"() -> (w672:string)
              n398 = local read "adccal"() -> (w669:string)
              n399 = global read "Test Parameter Globals_1.0.0.vi" "OperatorInfo"() -> (w675:string)
              n400 = call <vilib>:"Trim Whitespace.vi"("string"=w668) -> ("trimmed string"=w667:string)  [unwired: 1 in]
              n401 = local read "i_mon"() -> (w670:string)
              n402 = Concatenate Strings(w675, w660, w674, w673, w672, w671, w660, w670, w660, w669, w660, w667, w660, w662, w660, w661) -> (w666:string)
              n403 = call-poly <vilib>:"Read Delimited Spreadsheet.vi"("file path (dialog if empty)"=w663, "error in (no error)"=w665) -> ("new file path (Not A Path if cancelled)"=w682:path, "all rows"=w683:string[][], "error out"=w678:errorcluster)  [unwired: 8 in, 3 out]
              n404 = Build Array(w666) -> (w664:string[])
              n405 = Insert Into Array(array=w683, index (row)=0, new element=w664) -> (w680:string[][])  [unwired: 1 in]
              n406 = call-poly <vilib>:"Write Delimited Spreadsheet.vi"("file path (dialog if empty)"=w682, "2D data"=w680, "append to file? (new file:F)"=FALSE, "error in (no error)"=w678, "delimiter (\\t)"="," ("delimiter (\\t)")) -> ("error out"=w677:errorcluster)  [unwired: 9 in, 1 out]
            }
          }
        }
        frame True {
        }
      }
      n407 = local read "Status"() -> (w637:string)
      n408 = local read "Text"() -> (w635:refnum<vi>)
      n409 = call "BuildStrings_Return.vi"("seconds to wait"=1.0, "Input String"=w637, "New String"="DONE!!\n\nSetting up PNA...", "error in (no error)"=w643, "reference"=w635) -> ("error out"=w642:errorcluster, "concatenated string"=w636:string)  [unwired: 4 in, 1 out]
      n410 = local write "Status"(w636) -> ()
    }
    frame #13 {
      n411 = local read "Setup PNA (T)"() -> (w793:bool)
      n412 = global read "Station References Global.vi" "PNA Present?"() -> (w792:bool)
      n413 = And(x=w793, y=w792) -> (x .and. y?=w791:bool)
      n414 = case shown="True" w791 {
        tunnel: w788 -> [w796 w810]
        tunnel: [w796 w809] -> w790
        frame False {
        }
        frame True {
          w804 = 0 items=["Normal", "SMC"] ("MODE")
          w802 = 1 ("CH")
          w803 = i64 1000000000 items=["GHz"=1000000000, "MHZ"=1000000] ("Units")
          w818 = 1 ("Channel (1)")
          w817 = 1 ("Sweep Points (201)")
          w828 = 1 items=["Chopped", "Alternate"] ("Sweep Mode (0: Chopped)")
          w827 = 3 items=["Linear", "Logarithmic", "Power", "CW", "Segment", "Phase"] ("Sweep Type (0: Linear)")
          w826 = 1 ("Channel (1)")
          w822 = 3 items=["HOLD", "CONT", "GROUP", "SINGLE"]  # Mode
          w821 = 1  # Channel
          n415 = local read "PNA_STATE"() -> (w816:string)
          n416 = local read "Status"() -> (w811:string)
          n417 = Concatenate Strings("Loading PNA State ", w816) -> (w834:string)
          n418 = local read "Text"() -> (w812:refnum<vi>)
          n419 = global read "Station References Global.vi" "PNA"() -> (w829:refnum<visa-resource-name>)
          n420 = call "BuildStrings_Return.vi"("Input String"=w811, "New String"=w834, "error in (no error)"=w810, "reference"=w812) -> ("error out"=w820:errorcluster, "concatenated string"=w836:string)  [unwired: 5 in, 1 out]
          n421 = local write "Status"(w836) -> ()
          n422 = call "Recall.vi"("error in (no error)"=w820, "File Name ()"=w816, "VISA resource name"=w829) -> ("error out"=w799:errorcluster, "VISA resource name out"=w798:refnum<visa-resource-name>)  [unwired: 7 in]
          n423 = local read "REF_FREQ"() -> (w797:dbl)
          n424 = call "PNA-L_SET-CWFREQ.vi"("Session In"=w798, "error in"=w799, "MODE"=w804, "FREQ"=w797, "Units"=w803, "CH"=w802, "Source"=w802) -> ("Session Out"=w800:refnum<visa-resource-name>, "error out"=w801:errorcluster)  [unwired: 10 in, 1 out]
          n425 = call "Configure Sweep.vi"("Sweep Mode (0: Chopped)"=w828, "error in (no error)"=w801, "Sweep Type (0: Linear)"=w827, "Channel (1)"=w817, "VISA resource name"=w800) -> ("error out"=w833:errorcluster, "VISA resource name out"=w832:refnum<visa-resource-name>)  [unwired: 5 in]
          n426 = local read "REF_PWR"() -> (w819:dbl)
          n427 = call "Configure Sweep Generation.vi"("Sweep Points (201)"=w817, "error in (no error)"=w833, "Channel (1)"=w817, "VISA resource name"=w832) -> ("error out"=w814:errorcluster, "VISA resource name out"=w815:refnum<visa-resource-name>)  [unwired: 6 in]
          n428 = call "Configure Power.vi"("VISA resource name"=w815, "Enable RF Power (T: Enable)"=TRUE, "Channel (1)"=w818, "Port (1)"=w818, "error in (no error)"=w814, "Power Level (0 dBm)"=w819) -> ("VISA resource name out"=w805:refnum<visa-resource-name>, "error out"=w806:errorcluster)  [unwired: 8 in]
          n429 = call "Select Measurement.vi"("error in (no error)"=w806, "Measurement Name (CH1_S11_1)"="CH1_S11_1", "Channel (1)"=w826, "VISA resource name"=w805) -> ("error out"=w830:errorcluster, "VISA resource name out"=w831:refnum<visa-resource-name>)  [unwired: 6 in]
          n430 = call "Configure Marker_RageATE.vi"("Session In"=w831, "CH#"=w826, "MKR#"=1, "MKR ON(T)"=TRUE, "error in"=w830) -> ("Session Out"=w808:refnum<visa-resource-name>, "error out"=w807:errorcluster)  [unwired: 9 in]
          n431 = call "PNA_SWEEP MODE.vi"("Mode"=w822, "Channel"=w821, "error in (no error)"=w807, "VISA resource name"=w808) -> ("error out"=w809:errorcluster)  [unwired: 6 in, 1 out]
        }
      }
      n432 = local read "Status"() -> (w787:string)
      n433 = local read "Text"() -> (w786:refnum<vi>)
      n434 = call "BuildStrings_Return.vi"("Input String"=w787, "New String"="DONE!!!", "error in (no error)"=w790, "reference"=w786) -> ("error out"=w794:errorcluster, "concatenated string"=w789:string)  [unwired: 5 in, 1 out]
      n435 = local write "Status"(w789) -> ()
    }
    frame #14 {
      n436 = global read "Station References Global.vi" "Sig Gen1 Present?"() -> (w839:bool)
      n437 = case shown="True" w839 {
        tunnel: w838 -> [w840 w859]
        tunnel: [w840 w851] -> w837
        frame False {
        }
        frame True {
          n438 = local read "Status"() -> (w857:string)
          n439 = local read "Text"() -> (w856:refnum<vi>)
          n440 = local read "RF_POWER"() -> (w850:dbl)
          n441 = global read "Station References Global.vi" "SigGen1"() -> (w854:refnum<visa-resource-name>)
          n442 = call "BuildStrings_Return.vi"("Input String"=w857, "New String"="Setting up Sig Gen ...", "error in (no error)"=w859, "reference"=w856) -> ("error out"=w855:errorcluster, "concatenated string"=w841:string)  [unwired: 5 in, 1 out]
          n443 = local write "Status"(w841) -> ()
          n444 = call "VSG_SET-GET_AMPL_3.00.vi"("error in"=w855, "Set Power (num)"=w850, "Session In"=w854) -> ("error out"=w849:errorcluster, "Session Out"=w848:refnum<visa-resource-name>)  [unwired: 6 in, 1 out]
          n445 = call "VSG_SET_RF_STATE_1.00.vi"("RF ON/OFF (OFF)"=TRUE, "error in"=w849, "Session In"=w848) -> ("error out"=w843:errorcluster, "Session Out"=w846:refnum<visa-resource-name>)  [unwired: 6 in, 1 out]
          n446 = local read "RF_FREQ"() -> (w853:dbl)
          n447 = call "VISA_OPC.vi"("OPC(T)"=TRUE ("OPC?(T)"), "error in"=w843, "Session In"=w846) -> ("error out"=w844:errorcluster, "Session Out"=w845:refnum<visa-resource-name>)  [unwired: 6 in, 1 out]
          n448 = call "VSG_SET-GET_CW_1.00.vi"("Freq Units"="GHz", "error in"=w844, "Set Freq (MHz) num"=w853, "Session In"=w845) -> ("error out"=w851:errorcluster)  [unwired: 4 in, 3 out]
        }
      }
    }
    frame #15 {
      n449 = global read "Station References Global.vi" "Gantry Present?"() -> (w863:bool)
      n450 = local read "Setup Gantry(t)"() -> (w864:bool)
      n451 = And(x=w864, y=w863) -> (x .and. y?=w862:bool)
      n452 = case shown="True" w862 {
        tunnel: w861 -> [w865 w868]
        tunnel: [w865 w883] -> w860
        frame False {
        }
        frame True {
          w874 = u16 0 items=["Inches", "cm"] ("Zunits")
          n453 = global read "Station References Global.vi" "Gantry"() -> (w866:refnum<visa-resource-name>)
          n454 = for {
            N: 2 -> [_]
            tunnel: w866 -> [w893]
            shift-right: [w888] -> w869
            shift-left: w868 -> [w892]
            tunnel: [w885] -> _
            stop <- w886 stop-if-true
            w891 = TRUE ("Open Serial")
            n455 = call "WAM_ESS.vi"("VISA resource name"=w893, "error in (no error)"=w892, "Open Serial"=w891, "Test Running (T)"=w891, "Close Serial"=w891) -> ("Enabled(T-RO)"=w890:bool, "FH_NOT(T)"=w889:bool, "VISA resource name out"=w884:refnum<visa-resource-name>, "error out"=w887:errorcluster)  [unwired: 7 in]
            n456 = And(x=w890, y=w889) -> (x .and. y?=w886:bool)
            n457 = case shown="False" w886 {
              tunnel: [w902 w904] -> w888
              tunnel: w887 -> [w900 w904]
              tunnel: [w897 w903] -> w885
              tunnel: w884 -> [w896 w903]
              frame False {
                w894 = TRUE ("Close Serial")
                w895 = u16 1 items=["Disable Driver", "Enable Driver", "Read Driver Status"] ("Driver-Func")
                n458 = call "Prompt User for Input3"("error in (no error)"=w900) -> ("RESET"=w899:bool, "error out"=w901:errorcluster)  [unwired: 17 in]
                n459 = Not(x=w899) -> (.not. x?=w898:bool)
                n460 = Stop(stop? (T)=w898) -> ()
                n461 = call "Gantry_Driver.vi"("VISA resource name"=w896, "error in (no error)"=w901, "Open Serial"=w894, "Driver-Func"=w895, "Close Serial"=w894) -> ("VISA resource name out"=w897:refnum<visa-resource-name>, "error out"=w902:errorcluster)  [unwired: 11 in, 2 out]
              }
              frame True {
              }
            }
          }
          n462 = local read "Status"() -> (w881:string)
          n463 = local read "PORT"() -> (w871:i16)
          n464 = local read "Text"() -> (w880:refnum<vi>)
          n465 = local read "Gantry_Z"() -> (w873:dbl)
          n466 = global read "Station References Global.vi" "Gantry"() -> (w876:refnum<visa-resource-name>)
          n467 = call "BuildStrings_Return.vi"("Input String"=w881, "New String"="Setting up Gantry", "error in (no error)"=w869, "reference"=w880) -> ("error out"=w878:errorcluster, "concatenated string"=w877:string)  [unwired: 5 in, 1 out]
          n468 = Subtract(x=21, y=w871) -> (x-y=w870:i32)
          n469 = local write "Status"(w877) -> ()
          n470 = global write "Tetra_Globals.vi" "Gantry_Z"(w873) -> ()
          n471 = call "Gantry.vi"("COMPORT"=w876, "error in (no error)"=w878, "Antenna Select"=w870, "z ref"=21.0, "Write(reads antenna co-ords when off)"=TRUE, "z"=w873, "Zunits"=w874) -> ("error out"=w883:errorcluster)  [unwired: 12 in]
        }
      }
    }
    frame #16 {
      n472 = control-ref of="This VI"() -> (w915:refnum<vi>)
      n473 = property class="VI"(reference=w915) -> ("Path"=w913:path)  [unwired: 1 in, 2 out]
      n474 = local read "Status"() -> (w918:string)
      n475 = local read "Text"() -> (w917:refnum<vi>)
      n476 = Path To String(path=w913) -> (string=w914:string)
      n477 = call "BuildStrings_Return.vi"("seconds to wait"=2.0, "Input String"=w918, "New String"="Setup Complete !!!", "error in (no error)"=w916, "reference"=w917) -> ("error out"=w906:errorcluster, "concatenated string"=w908:string)  [unwired: 4 in, 1 out]
      n478 = Search and Replace String(input string=w914, search string=".vi", replace string=".txt" ("replace string (\"\")")) -> (result string=w909:string)  [unwired: 5 in, 3 out]
      n479 = local write "Status"(w908) -> ()
      n480 = String To Path(string=w909) -> (path=w910:path)
      n481 = Build Array(w908) -> (w907:string[])
      n482 = call-poly <vilib>:"Write Delimited Spreadsheet.vi"("file path (dialog if empty)"=w910, "1D data"=w907, "error in (no error)"=w906) -> ("error out"=w905:errorcluster)  [unwired: 11 in, 1 out]
    }
  }
  "error out" <- w12
